vi "EnvFindModel.vi"(11 "Env String":string) -> (3 "Enum":enum16{"TEMP2700", "2416", ""}(ring))   [LabVIEW 2016]
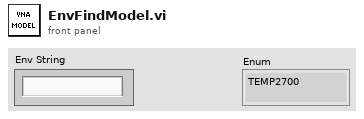
[diagram p1: front panel]
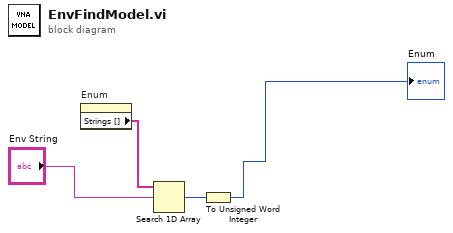
[diagram p0: block diagram]
diagram:
  n1 = property on="Enum" class="Enum (strict)"() -> ("Strings []"=w4:string[])  [unwired: 2 in, 2 out]
  n2 = Search 1D Array(1D array=w4, element="Env String") -> (index of element=w2:i32)  [unwired: 1 in]
  n3 = To Unsigned Word Integer(number=w2) -> (unsigned 16bit integer=→"Enum":u16)
